vi "_builtins_connect_pane.vi"(8 "error in (no error)":errorcluster, 11 "VI Refnum in":refnum<vi>) -> (0 "error out":errorcluster, 3 "VI Refnum out":refnum<vi>)   [LabVIEW 2019, in "Script.lvlib"]
doc: "Wires the selected front panel controls and indicators to the connector pane ordered top-to-bottom then left-to-right respectively. Error In and Error Out terminals are wired to the bottom-left and bottom-right. All control terminals are set to Required inputs.\n\nCreated by: Ryan Pacini"
uses:
  Script.lvlib
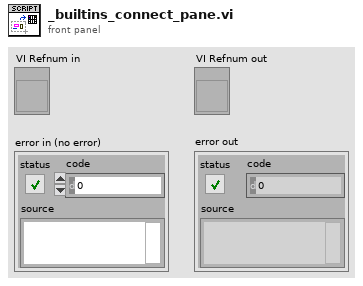
[diagram p1: front panel]
types:
  T1 = cluster{"Top":i16, "Left":i16, "Control":refnum<vi>}
  T2 = enum16{"Invalid Wire Rule", "Required", "Recommended", "Optional", "Dynamic Dispatch"}
  T3 = typedef "LVRectTypeDef.ctl" = cluster{"Left":i16, "Top":i16, "Right":i16, "Bottom":i16}
  T4 = cluster{"Top":i16, "Left":i16, "Control":refnum<vi>}[]
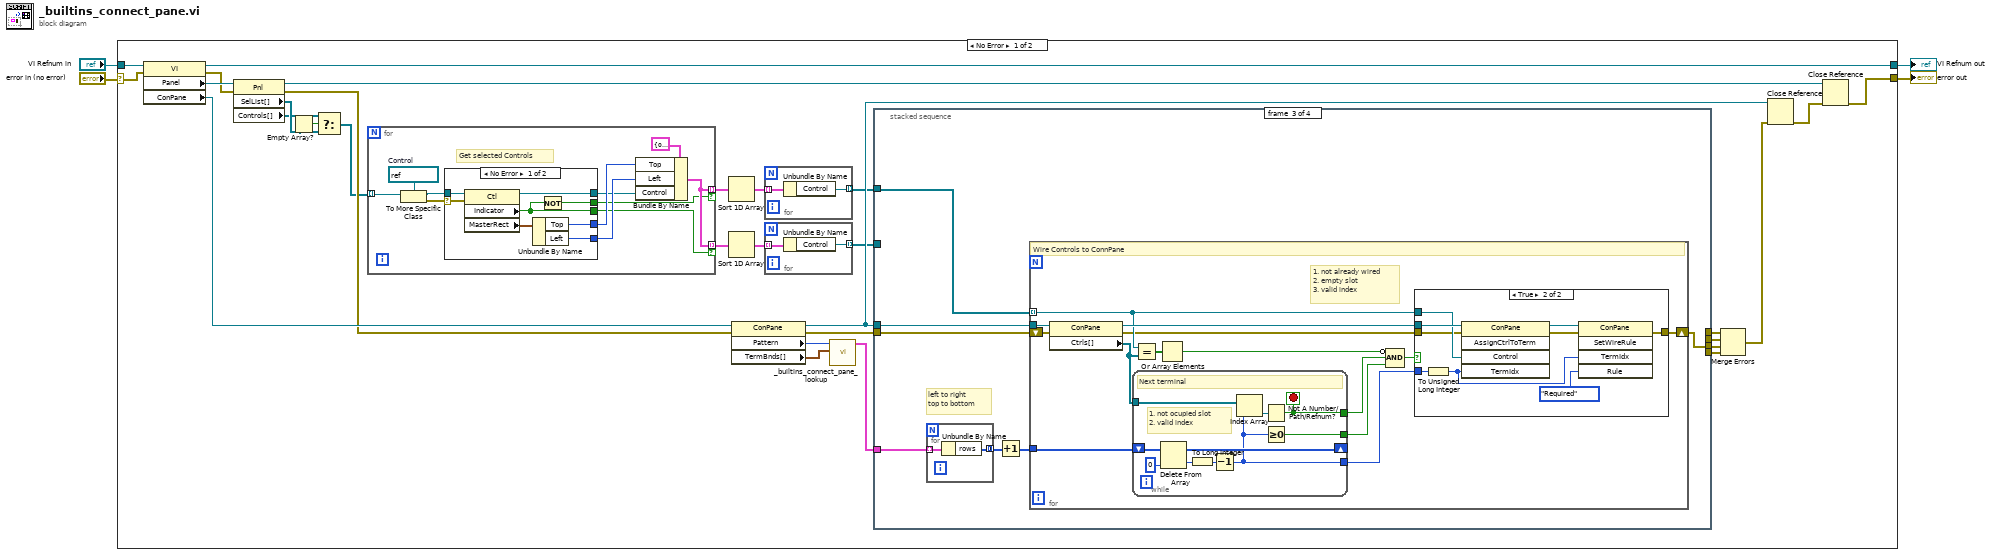
[diagram p0: block diagram]
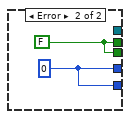
[diagram p2: hidden frame]
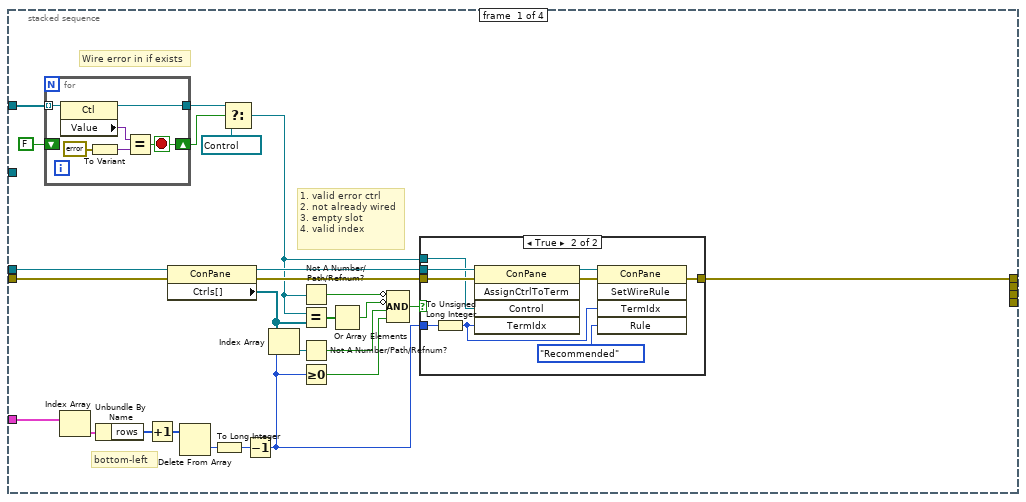
[diagram p3: hidden frame]
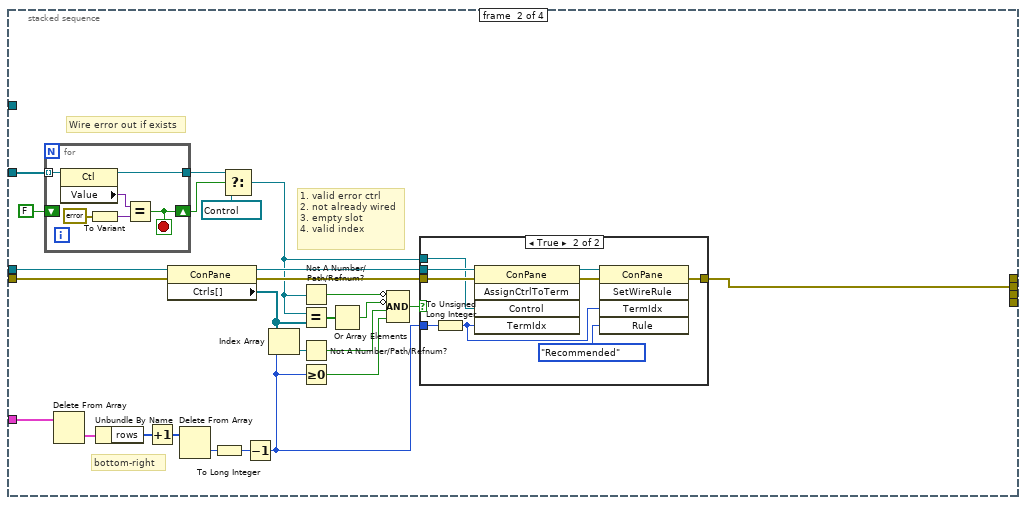
[diagram p5: hidden frame]
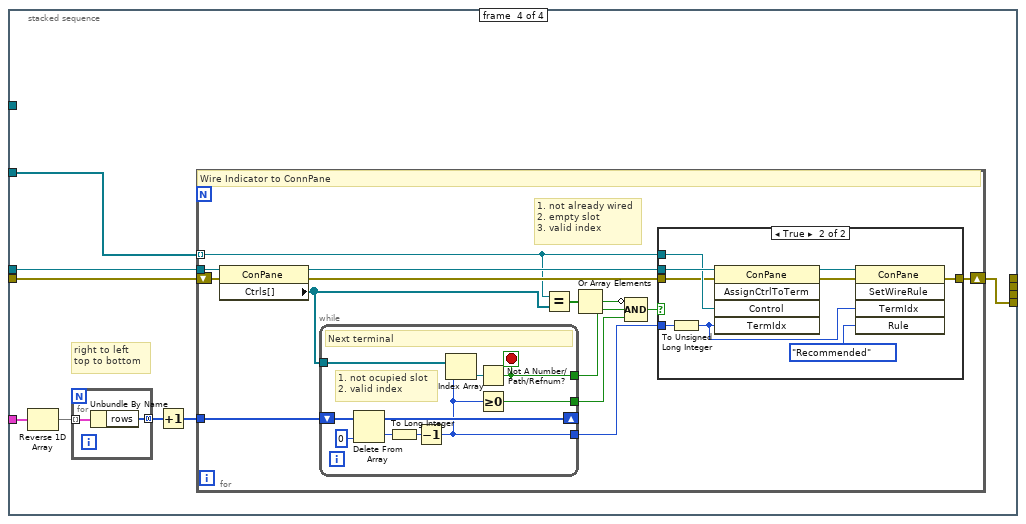
[diagram p8: hidden frame]
diagram:
  n1 = case shown="No Error" "error in (no error)" {
    selector: "error in (no error)" -> [w33 w231]
    tunnel: [w30 w232] -> w4
    tunnel: "VI Refnum in" -> [w34 w232]
    tunnel: [w15 w231] -> w1
    frame No Error {
      n2 = property on="Property Node" class="VI"(reference=w34, error in=w33) -> (reference out=w30:refnum<vi>, error out=w31:errorcluster, "Panel"=w32:refnum<vi>, "ConPane"=w25:refnum<vi>)
      n3 = property on="Property Node" class="Pnl"(reference=w32, error in=w31) -> (reference out=w17:refnum<vi>, error out=w22:errorcluster, "SelList[]"=w7:refnum<vi>[], "Controls[]"=w6:refnum<vi>[])
      n4 = Empty Array?(array=w7) -> (empty?=w8:bool)
      n5 = Select(t=w6, s=w8, f=w7) -> (s? t:f=w5:refnum<vi>[])
      n6 = for {
        tunnel: w5 -> [w49] mode=indexing
        tunnel: [w44] -> w29 mode=indexing if=w41
        tunnel: [w44] -> w28 mode=indexing if=w40
        w48 = refnum<vi> refnum  # Control
        # "Get selected Controls"
        n7 = To More Specific Class(target class=w48, reference=w49) -> (specific class reference=w46:refnum<vi>, error out=w47:errorcluster)  [unwired: 1 in]
        n8 = case shown="No Error" w47 {
          selector: w47 -> [w50 _]
          tunnel: w46 -> [w57 _]
          tunnel: [w53 w59] -> w40
          tunnel: [w55 _] -> w39
          tunnel: [w54 w58] -> w45
          tunnel: [w52 w59] -> w41
          tunnel: [w51 w58] -> w42
          frame No Error {
            n9 = property class="Ctl"(reference=w57, error in=w50) -> (reference out=w55:refnum<vi>, "Indicator"=w53:bool, "MasterRect"=w56:T3)  [unwired: 1 out]
            n10 = Unbundle By Name(w56) -> ("Top"=w54:i16, "Left"=w51:i16)
            n11 = Not(x=w53) -> (.not. x?=w52:bool)
          }
          frame Error {
            w58 = i16 0 ("Top")
            w59 = FALSE
          }
        }
        n12 = Bundle By Name(cluster=T1 {"Top"=0, "Left"=0, "Control"=refnum}, "Top"=w45, "Left"=w42, "Control"=w39) -> (w44:T1)
      }
      n13 = Sort 1D Array(array=w29) -> (sorted array=w14:T4)
      n14 = Sort 1D Array(array=w28) -> (sorted array=w12:T4)
      n15 = property class="ConPane"(reference=w25, error in=w22) -> (reference out=w18:refnum<vi>, error out=w23:errorcluster, "Pattern"=w27:u32, "TermBnds[]"=w26:T3[])
      n16 = for {
        tunnel: w14 -> [w38] mode=indexing
        tunnel: [w37] -> w13 mode=indexing
        n17 = Unbundle By Name(w38) -> ("Control"=w37:refnum<vi>)
      }
      n18 = for {
        tunnel: w12 -> [w36] mode=indexing
        tunnel: [w35] -> w11 mode=indexing
        n19 = Unbundle By Name(w36) -> ("Control"=w35:refnum<vi>)
      }
      n20 = call "_builtins_connect_pane_lookup.vi"("TermBnds"=w26, "Pattern"=w27) -> ("columns"=w24:cluster{"rows":u8[]}[])  [unwired: 9 in]
      n21 = stacked-sequence {
        tunnel: w13 -> [w82 _ w145 _]
        tunnel: w24 -> [w64 w105 w150 w194]
        tunnel: w18 -> [w71 w115 w149 w193]
        tunnel: w11 -> [_ w103 _ w188]
        tunnel: w23 -> [w73 w116 w147 w191]
        tunnel: [_ _ w146 _] -> w21
        tunnel: [_ _ _ w187] -> w20
        tunnel: [_ w102 _ _] -> w10
        tunnel: [w60 _ _ _] -> w9
        frame #0 {
          # "bottom-left"
          # "1. valid error ctrl\n2. not already wired\n3. empty slot\n4. valid index"
          # "Wire error in if exists"
          n22 = for {
            tunnel: w82 -> [w101] mode=indexing
            tunnel: [w97] -> w84
            shift-right: [w96] -> w85
            shift-left: FALSE -> [_]
            stop <- w96 stop-if-true
            n23 = property class="Ctl"(reference=w101) -> (reference out=w97:refnum<vi>, "Value"=w100:variant)  [unwired: 1 in, 1 out]
            n24 = To Variant(anything=errorcluster {"status"=FALSE, "code"=0, "source"=""} ("error in (no error)")) -> (Variant=w98:variant)
            n25 = Equal?(x=w100, y=w98) -> (x = y?=w96:bool)
          }
          n26 = Index Array(array=w64) -> (element=w72:cluster{"rows":u8[]})  [unwired: 1 in]
          n27 = Unbundle By Name(w72) -> ("rows"=w66:u8[])
          n28 = Increment(x=w66) -> (x+1=w63:u8[])
          n29 = property class="ConPane"(reference=w71, error in=w73) -> (reference out=w70:refnum<vi>, error out=w69:errorcluster, "Ctrls[]"=w77:refnum<vi>[])
          n30 = Delete From Array(array=w63) -> (deleted portion=w79:u8)  [unwired: 2 in, 1 out]
          n31 = To Long Integer(number=w79) -> (32bit integer=w65:i32)
          n32 = Select(t=w84, s=w85, f=refnum<vi> refnum) -> (s? t:f=w62:refnum<vi>)
          n33 = Decrement(x=w65) -> (x-1=w68:i32)
          n34 = Index Array(array=w77, index=w68) -> (element=w80:refnum<vi>)
          n35 = Not A Number/Path/Refnum?(number/path/refnum=w62) -> (NaN/Path/Refnum?=w61:bool)
          n36 = Equal?(x=w62, y=w77) -> (x = y?=w76:bool[])
          n37 = Not A Number/Path/Refnum?(number/path/refnum=w80) -> (NaN/Path/Refnum?=w78:bool)
          n38 = Greater Or Equal To 0?(x=w68) -> (x >= 0?=w74:bool)
          n39 = Or Array Elements(Boolean array=w76) -> (logical OR=w75:bool)
          n40 = Compound Arithmetic op=AND(invert w61, invert w75, w78, w74) -> (w67:bool)
          n41 = case shown="True" w67 {
            tunnel: w70 -> [_ w95]
            tunnel: w69 -> [w86 w94]
            tunnel: w68 -> [_ w93]
            tunnel: w62 -> [_ w92]
            tunnel: [w86 w89] -> w60
            frame False {
            }
            frame True {
              n42 = To Unsigned Long Integer(number=w93) -> (unsigned 32bit integer=w88:u32)
              n43 = invoke class="ConPane" method="AssignCtrlToTerm"(reference=w95, error in=w94, "Control"=w92, "TermIdx"=w88) -> (reference out=w91:refnum<vi>, error out=w90:errorcluster)  [unwired: 1 in, 3 out]
              n44 = invoke class="ConPane" method="SetWireRule"(reference=w91, error in=w90, "TermIdx"=w88, "Rule"=T2."Recommended") -> (error out=w89:errorcluster)  [unwired: 1 in, 4 out]
            }
          }
        }
        frame #1 {
          # "bottom-right"
          # "1. valid error ctrl\n2. not already wired\n3. empty slot\n4. valid index"
          # "Wire error out if exists"
          n45 = for {
            tunnel: w103 -> [w143] mode=indexing
            tunnel: [w139] -> w126
            shift-right: [w138] -> w127
            shift-left: FALSE -> [_]
            stop <- w138 stop-if-true
            n46 = property class="Ctl"(reference=w143) -> (reference out=w139:refnum<vi>, "Value"=w142:variant)  [unwired: 1 in, 1 out]
            n47 = To Variant(anything=errorcluster {"status"=FALSE, "code"=0, "source"=""} ("error in (no error)")) -> (Variant=w140:variant)
            n48 = Equal?(x=w142, y=w140) -> (x = y?=w138:bool)
          }
          n49 = Delete From Array(array=w105) -> (deleted portion=w104:cluster{"rows":u8[]})  [unwired: 2 in, 1 out]
          n50 = Unbundle By Name(w104) -> ("rows"=w110:u8[])
          n51 = Increment(x=w110) -> (x+1=w108:u8[])
          n52 = property class="ConPane"(reference=w115, error in=w116) -> (reference out=w114:refnum<vi>, error out=w113:errorcluster, "Ctrls[]"=w120:refnum<vi>[])
          n53 = Delete From Array(array=w108) -> (deleted portion=w122:u8)  [unwired: 2 in, 1 out]
          n54 = To Long Integer(number=w122) -> (32bit integer=w109:i32)
          n55 = Select(t=w126, s=w127, f=refnum<vi> refnum) -> (s? t:f=w107:refnum<vi>)
          n56 = Decrement(x=w109) -> (x-1=w112:i32)
          n57 = Index Array(array=w120, index=w112) -> (element=w123:refnum<vi>)
          n58 = Not A Number/Path/Refnum?(number/path/refnum=w107) -> (NaN/Path/Refnum?=w106:bool)
          n59 = Equal?(x=w107, y=w120) -> (x = y?=w119:bool[])
          n60 = Not A Number/Path/Refnum?(number/path/refnum=w123) -> (NaN/Path/Refnum?=w121:bool)
          n61 = Greater Or Equal To 0?(x=w112) -> (x >= 0?=w117:bool)
          n62 = Or Array Elements(Boolean array=w119) -> (logical OR=w118:bool)
          n63 = Compound Arithmetic op=AND(invert w106, invert w118, w121, w117) -> (w111:bool)
          n64 = case shown="True" w111 {
            tunnel: w114 -> [_ w137]
            tunnel: w113 -> [w128 w136]
            tunnel: w112 -> [_ w135]
            tunnel: w107 -> [_ w134]
            tunnel: [w128 w132] -> w102
            frame False {
            }
            frame True {
              n65 = To Unsigned Long Integer(number=w135) -> (unsigned 32bit integer=w129:u32)
              n66 = invoke class="ConPane" method="AssignCtrlToTerm"(reference=w137, error in=w136, "Control"=w134, "TermIdx"=w129) -> (reference out=w131:refnum<vi>, error out=w133:errorcluster)  [unwired: 1 in, 3 out]
              n67 = invoke class="ConPane" method="SetWireRule"(reference=w131, error in=w133, "TermIdx"=w129, "Rule"=T2."Recommended") -> (error out=w132:errorcluster)  [unwired: 1 in, 4 out]
            }
          }
        }
        frame #2 {
          # "left to right\ntop to bottom"
          n68 = for {
            tunnel: w150 -> [w186] mode=indexing
            tunnel: [w185] -> w144 mode=concatenating
            n69 = Unbundle By Name(w186) -> ("rows"=w185:u8[])
          }
          n70 = Increment(x=w144) -> (x+1=w148:u8[])
          n71 = for {
            tunnel: w145 -> [w160] mode=indexing
            shift-right: [w156] -> w146
            shift-left: w147 -> [w155]
            tunnel: w149 -> [w164]
            tunnel: w148 -> [w163]
            # "1. not already wired\n2. empty slot\n3. valid index"
            # "Wire Controls to ConnPane"
            n72 = property class="ConPane"(reference=w164, error in=w155) -> (reference out=w162:refnum<vi>, error out=w157:errorcluster, "Ctrls[]"=w151:refnum<vi>[])
            n73 = while {
              tunnel: [w169] -> w154
              tunnel: [w165] -> w153
              tunnel: [w167] -> w152
              tunnel: w151 -> [w166]
              shift-right: [w172] -> _
              shift-left: w163 -> [w174]
              stop <- w165 stop-if-true
              # "1. not ocupied slot\n2. valid index"
              # "Next terminal"
              n74 = Delete From Array(array=w174, index=0) -> (deleted portion=w170:u8, array with subset deleted=w172:u8[])  [unwired: 1 in]
              n75 = To Long Integer(number=w170) -> (32bit integer=w168:i32)
              n76 = Decrement(x=w168) -> (x-1=w169:i32)
              n77 = Index Array(array=w166, index=w169) -> (element=w171:refnum<vi>)
              n78 = Not A Number/Path/Refnum?(number/path/refnum=w171) -> (NaN/Path/Refnum?=w165:bool)
              n79 = Greater Or Equal To 0?(x=w169) -> (x >= 0?=w167:bool)
            }
            n80 = Equal?(x=w160, y=w151) -> (x = y?=w159:bool[])
            n81 = Or Array Elements(Boolean array=w159) -> (logical OR=w158:bool)
            n82 = Compound Arithmetic op=AND(invert w158, w153, w152) -> (w161:bool)
            n83 = case shown="True" w161 {
              tunnel: w162 -> [_ w184]
              tunnel: w160 -> [_ w183]
              tunnel: w154 -> [_ w182]
              tunnel: w157 -> [w175 w181]
              tunnel: [w175 w178] -> w156
              frame False {
              }
              frame True {
                n84 = To Unsigned Long Integer(number=w182) -> (unsigned 32bit integer=w176:u32)
                n85 = invoke class="ConPane" method="AssignCtrlToTerm"(reference=w184, error in=w181, "Control"=w183, "TermIdx"=w176) -> (reference out=w177:refnum<vi>, error out=w179:errorcluster)  [unwired: 1 in, 3 out]
                n86 = invoke class="ConPane" method="SetWireRule"(reference=w177, error in=w179, "TermIdx"=w176, "Rule"=T2."Required") -> (error out=w178:errorcluster)  [unwired: 1 in, 4 out]
              }
            }
          }
        }
        frame #3 {
          # "right to left\ntop to bottom"
          n87 = Reverse 1D Array(array=w194) -> (reversed array=w189:cluster{"rows":u8[]}[])
          n88 = for {
            tunnel: w189 -> [w230] mode=indexing
            tunnel: [w229] -> w190 mode=concatenating
            n89 = Unbundle By Name(w230) -> ("rows"=w229:u8[])
          }
          n90 = Increment(x=w190) -> (x+1=w192:u8[])
          n91 = for {
            tunnel: w188 -> [w198] mode=indexing
            shift-right: [w195] -> w187
            shift-left: w191 -> [w204]
            tunnel: w193 -> [w208]
            tunnel: w192 -> [w207]
            # "1. not already wired\n2. empty slot\n3. valid index"
            # "Wire Indicator to ConnPane"
            n92 = property class="ConPane"(reference=w208, error in=w204) -> (reference out=w199:refnum<vi>, error out=w200:errorcluster, "Ctrls[]"=w201:refnum<vi>[])
            n93 = while {
              tunnel: [w223] -> w196
              tunnel: [w219] -> w203
              tunnel: [w221] -> w202
              tunnel: w201 -> [w220]
              shift-right: [w226] -> _
              shift-left: w207 -> [w228]
              stop <- w219 stop-if-true
              # "1. not ocupied slot\n2. valid index"
              # "Next terminal"
              n94 = Delete From Array(array=w228, index=0) -> (deleted portion=w224:u8, array with subset deleted=w226:u8[])  [unwired: 1 in]
              n95 = To Long Integer(number=w224) -> (32bit integer=w222:i32)
              n96 = Decrement(x=w222) -> (x-1=w223:i32)
              n97 = Index Array(array=w220, index=w223) -> (element=w225:refnum<vi>)
              n98 = Not A Number/Path/Refnum?(number/path/refnum=w225) -> (NaN/Path/Refnum?=w219:bool)
              n99 = Greater Or Equal To 0?(x=w223) -> (x >= 0?=w221:bool)
            }
            n100 = Equal?(x=w198, y=w201) -> (x = y?=w206:bool[])
            n101 = Or Array Elements(Boolean array=w206) -> (logical OR=w205:bool)
            n102 = Compound Arithmetic op=AND(invert w205, w203, w202) -> (w197:bool)
            n103 = case shown="True" w197 {
              tunnel: w199 -> [_ w218]
              tunnel: w198 -> [_ w217]
              tunnel: w196 -> [_ w216]
              tunnel: w200 -> [w209 w215]
              tunnel: [w209 w212] -> w195
              frame False {
              }
              frame True {
                n104 = To Unsigned Long Integer(number=w216) -> (unsigned 32bit integer=w210:u32)
                n105 = invoke class="ConPane" method="AssignCtrlToTerm"(reference=w218, error in=w215, "Control"=w217, "TermIdx"=w210) -> (reference out=w211:refnum<vi>, error out=w213:errorcluster)  [unwired: 1 in, 3 out]
                n106 = invoke class="ConPane" method="SetWireRule"(reference=w211, error in=w213, "TermIdx"=w210, "Rule"=T2."Recommended") -> (error out=w212:errorcluster)  [unwired: 1 in, 4 out]
              }
            }
          }
        }
      }
      n107 = Merge Errors(w9, w10, w21, w20) -> (w19:errorcluster)
      n108 = Close Reference(reference=w18, error in (no error)=w19) -> (error out=w16:errorcluster)
      n109 = Close Reference(reference=w17, error in (no error)=w16) -> (error out=w15:errorcluster)
    }
    frame Error {
    }
  }
  "VI Refnum out" <- w4
  "error out" <- w1
